vi "Memory Leak Tester.vi"() -> (0 "error out":errorcluster, 3 "ACNET Device Readings":T1(array[cluster]))   [LabVIEW 2013]
uses:
  <vilib>/httpClient/LabVIEWHTTPClient.lvlib
panel:
  in  "url":string="http://www-bd.fnal.gov/getdaq/job/$(DEVICE_LIST)?type=xml&iso-time=true&quiet=true"
  in  "stop":bool
  in  "Devices":string[](array[string])
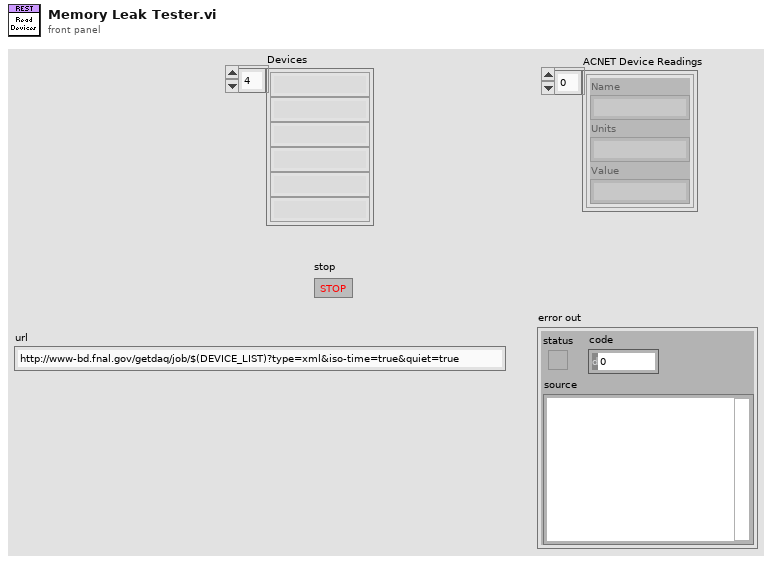
[diagram p1: front panel]
types:
  T1 = cluster{"Name":string, "Units":string, "Value":string}[]
  T2 = typedef "LabVIEWHTTPClient.lvlib/ClientHandle.ctl" = refnum<k1>
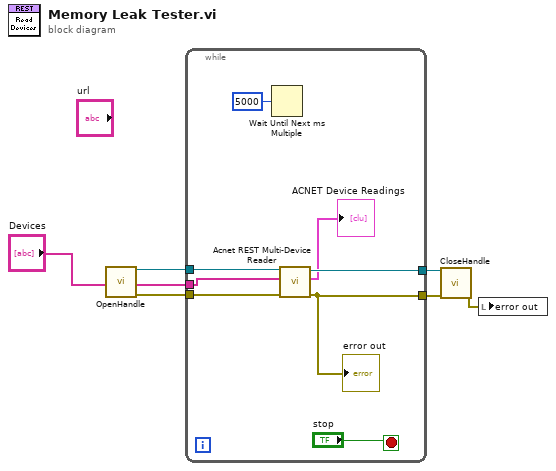
[diagram p0: block diagram]
diagram:
  n1 = call <vilib>:"OpenHandle.vi"() -> ("client handle out"=w5:T2, "error out"=w4:errorcluster)  [unwired: 14 in]
  n2 = while {
    tunnel: [w8] -> w2
    tunnel: "Devices" -> [w12]
    tunnel: w5 -> [w11]
    tunnel: w4 -> [w10]
    tunnel: [w9] -> w3
    stop <- "stop" stop-if-true
    n3 = Wait Until Next ms Multiple(millisecond multiple=u32 5000) -> ()  [unwired: 1 out]
    n4 = call "Acnet REST Multi-Device Reader.vi"("error in (no error)"=w10, "Devices"=w12, "client handle"=w11) -> ("error out"=w8:errorcluster, "ACNET Device Readings"=→"ACNET Device Readings":T1, "client handle out"=w9:T2)  [unwired: 6 in]
    "error out" <- w8
  }
  n5 = call <vilib>:"CloseHandle.vi"("client handle"=w3, "error in (no error)"=w2) -> ("error out"=w1:errorcluster)  [unwired: 13 in]
  n6 = local write "error out"(w1) -> ()
